vi "Untitled 1.vi"   [LabVIEW 2020]
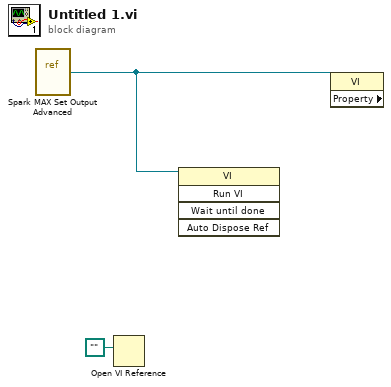
[diagram p0: block diagram]
diagram:
  n1 = vi-ref <vilib>:"Spark MAX Set Output Advanced.vi"() -> (w1:refnum<vi>)
  n2 = Open VI Reference(vi path=path "") -> ()  [unwired: 5 in, 2 out]
  n3 = invoke class="VI" method="Run VI"(reference=w1) -> ()  [unwired: 4 in, 5 out]
  n4 = property class="VI" props=[](reference=w1) -> ()  [unwired: 1 in, 3 out]
